vi "WLAN Rx Test Get RfsgWlan Handle.vi"(8 "error in (no error)":errorcluster, 11 "WLAN Tx Test in":refnum<class "niDTS WLAN Rx Test.lvclass">) -> (0 "error out":errorcluster, 2 "niRfsgWlan Handles":T1[][](array[typedef]), 3 "WLAN Tx Test out":refnum<class "niDTS WLAN Rx Test.lvclass">)   [LabVIEW 2015, in "niDTS WLAN.lvlib" / "niDTS WLAN Rx Test.lvclass"]
uses:
  niDTS WLAN Rx Test.lvclass
  RiviInstDriver/niRfsgWlan/Includes/niRfsgWlan INC Handle.ctl
  RiviInstDriver/niRfsgWlan/Objects/niRfsgWlan.lvclass
  niDTS WLAN Rx Test.lvclass/niDTS WLAN Rx Test.ctl
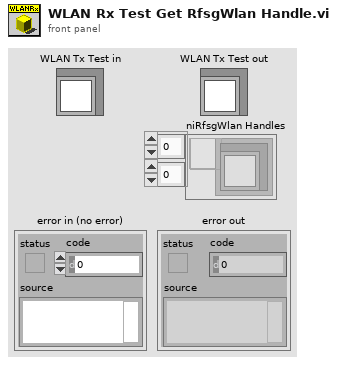
[diagram p1: front panel]
types:
  T1 = typedef "niRfsgWlan.lvclass/niRfsgWlan INC Handle.ctl" = refnum<data-value>
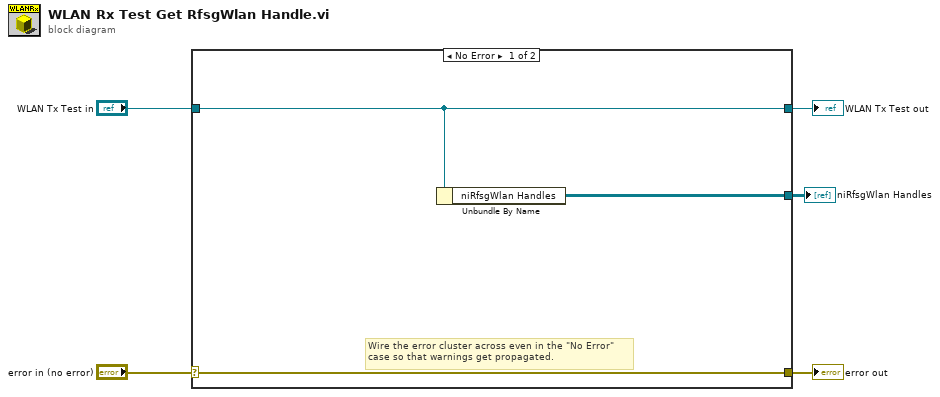
[diagram p0: block diagram]
diagram:
  n1 = case shown="No Error" "error in (no error)" {
    selector: "error in (no error)" -> [w8 w10]
    tunnel: [w8 w10] -> w4
    tunnel: [w7 w9] -> w2
    tunnel: "WLAN Tx Test in" -> [w7 w9]
    tunnel: [w6 _] -> w1
    frame No Error {
      # "Wire the error cluster across even in the \"No Error\"\ncase so that warnings get propagated."
      n2 = Unbundle By Name(w7) -> ("niRfsgWlan Handles"=w6:T1[][])
    }
    frame Error {
    }
  }
  "error out" <- w4
  "WLAN Tx Test out" <- w2
  "niRfsgWlan Handles" <- w1
